vi "Vin_Vout_DCDIFF.vi"(0 "V in volt":dbl format="%0.2f", 1 "Fondo Scala AI0 (68-34)":dbl(ring)=10.0 items=["10"=10.0, "5"=5.0, "0.5"=0.5, "0.05"=0.05], 2 "Fondo Scala AI1 (33)":dbl(ring)=10.0 items=["10"=10.0, "5"=5.0, "0.5"=0.5, "0.05"=0.05]) -> (3 "V0 medio":dbl format="%.5f", 4 "sd 0":dbl format="%.5f", 5 "V1 medio":dbl format="%.5f", 6 "sd 1":dbl format="%.5f")   [LabVIEW 2014]
uses:
  <vilib>/DAQmx/write.llb/DAQmx Write (Analog DBL 1Chan 1Samp).vi
  <vilib>/DAQmx/read.llb/DAQmx Read (Analog 1D DBL 1Chan NSamp).vi
  <vilib>/DAQmx/create/channels.llb/DAQmx Create Channel (AO-Voltage-Basic).vi
  <vilib>/DAQmx/configure/timing.llb/DAQmx Timing (Sample Clock).vi
  <vilib>/DAQmx/miscellaneous.llb/DAQmx Fill In Error Info.vi
  <vilib>/DAQmx/create/channels.llb/DAQmx Create Channel (AI-Voltage-Basic).vi
  <vilib>/Analysis/NI_AALBase.lvlib
panel:
  # "DIFFERENTIAL: 68 34\nRSE: 33"
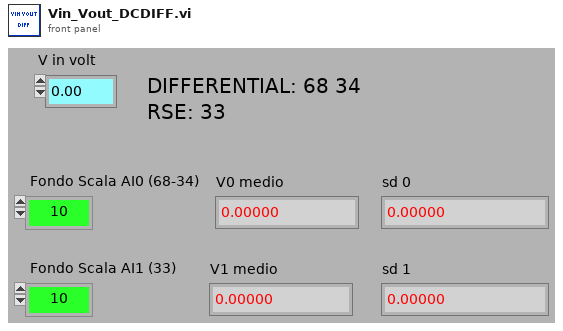
[diagram p1: front panel]
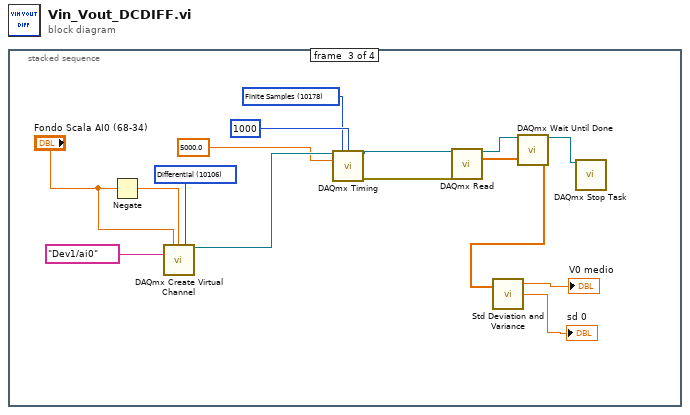
[diagram p0: block diagram]
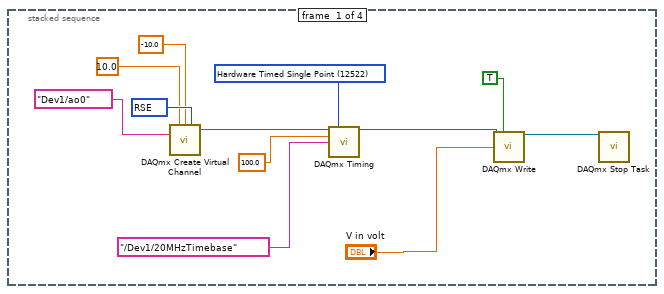
[diagram p2: hidden frame]
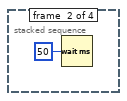
[diagram p3: hidden frame]
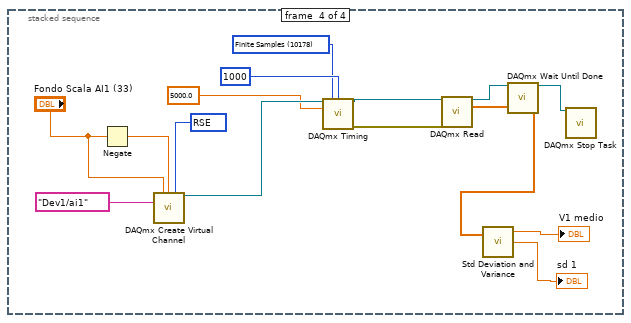
[diagram p4: hidden frame]
diagram:
  n1 = stacked-sequence {
    frame #0 {
      w8 = 12522 items=["Finite Samples"=10178, "Continuous Samples"=10123, "Hardware Timed Single Point"=12522] ("sample mode")
      w12 = 10083 items=["Default"=-1, "RSE"=10083, "Differential"=10106, "Pseudodifferential"=12529] ("output terminal configuration")
      n2 = call-poly <vilib>:"DAQmx Create Virtual Channel.vi"("maximum value"=10.0, "minimum value"=-10.0, "output terminal configuration"=w12, "physical channels"=tag "Dev1/ao0" ("Canale uscita")) -> ("task out"=w4:refnum<k21>)  [unwired: 5 in, 6 out]
      n3 = call-poly <vilib>:"DAQmx Timing.vi"("task/channels in"=w4, "sample mode"=w8, "rate"=100.0, "source"=tag "/Dev1/20MHzTimebase") -> ("task out"=w6:refnum<k21>)  [unwired: 3 in, 8 out]
      n4 = call-poly <vilib>:"DAQmx Write.vi"("task/channels in"=w6, "auto start"=TRUE, "data"="V in volt") -> ("task out"=w5:refnum<k21>)  [unwired: 1 in, 11 out]
      n5 = call <vilib>:"DAQmx Stop Task.vi"("task/channels in"=w5) -> ()  [unwired: 1 in, 14 out]
    }
    frame #1 {
      n6 = Wait (ms)(milliseconds to wait=u32 50) -> ()  [unwired: 1 out]
    }
    frame #2 {
      w19 = 10178 items=["Finite Samples"=10178, "Continuous Samples"=10123, "Hardware Timed Single Point"=12522] ("sample mode")
      w27 = 10106 items=["default"=-1, "RSE"=10083, "NRSE"=10078, "Differential"=10106, "Pseudodifferential"=12529] ("input terminal configuration")
      n7 = Negate(x="Fondo Scala AI0 (68-34)") -> (-x=w28:dbl)
      n8 = call-poly <vilib>:"DAQmx Create Virtual Channel.vi"("maximum value"="Fondo Scala AI0 (68-34)", "minimum value"=w28, "input terminal configuration"=w27, "physical channels"=tag "Dev1/ai0") -> ("task out"=w22:refnum<k21>)  [unwired: 5 in, 6 out]
      n9 = call-poly <vilib>:"DAQmx Timing.vi"("task/channels in"=w22, "sample mode"=w19, "samples per channel"=u32 1000, "rate"=5000.0) -> ("task out"=w25:refnum<k21>, "error out"=w24:errorcluster)  [unwired: 3 in, 7 out]
      n10 = call-poly <vilib>:"DAQmx Read.vi"("task/channels in"=w25, "error in"=w24) -> ("task out"=w20:refnum<k21>, "data"=w17:dbl[])  [unwired: 1 in, 11 out]
      n11 = call <vilib>:"Std Deviation and Variance.vi"("X"=w17) -> ("mean"=→"V0 medio":dbl, "standard deviation"=→"sd 0":dbl)  [unwired: 1 in, 1 out]
      n12 = call <vilib>:"DAQmx Wait Until Done.vi"("task/channels in"=w20) -> ("task out"=w18:refnum<k21>)  [unwired: 2 in, 12 out]
      n13 = call <vilib>:"DAQmx Stop Task.vi"("task/channels in"=w18) -> ()  [unwired: 1 in, 14 out]
    }
    frame #3 {
      w34 = 10178 items=["Finite Samples"=10178, "Continuous Samples"=10123, "Hardware Timed Single Point"=12522] ("sample mode")
      w42 = 10083 items=["default"=-1, "RSE"=10083, "NRSE"=10078, "Differential"=10106, "Pseudodifferential"=12529] ("input terminal configuration")
      n14 = Negate(x="Fondo Scala AI1 (33)") -> (-x=w43:dbl)
      n15 = call-poly <vilib>:"DAQmx Create Virtual Channel.vi"("maximum value"="Fondo Scala AI1 (33)", "minimum value"=w43, "input terminal configuration"=w42, "physical channels"=tag "Dev1/ai1") -> ("task out"=w37:refnum<k21>)  [unwired: 5 in, 6 out]
      n16 = call-poly <vilib>:"DAQmx Timing.vi"("task/channels in"=w37, "sample mode"=w34, "samples per channel"=u32 1000, "rate"=5000.0) -> ("task out"=w40:refnum<k21>, "error out"=w39:errorcluster)  [unwired: 3 in, 7 out]
      n17 = call-poly <vilib>:"DAQmx Read.vi"("task/channels in"=w40, "error in"=w39) -> ("task out"=w35:refnum<k21>, "data"=w32:dbl[])  [unwired: 1 in, 11 out]
      n18 = call <vilib>:"Std Deviation and Variance.vi"("X"=w32) -> ("mean"=→"V1 medio":dbl, "standard deviation"=→"sd 1":dbl)  [unwired: 1 in, 1 out]
      n19 = call <vilib>:"DAQmx Wait Until Done.vi"("task/channels in"=w35) -> ("task out"=w33:refnum<k21>)  [unwired: 2 in, 12 out]
      n20 = call <vilib>:"DAQmx Stop Task.vi"("task/channels in"=w33) -> ()  [unwired: 1 in, 14 out]
    }
  }
